vi "DAQmx Create Channel (CO-Pulse Generation-Frequency).vi"(0 "task in":refnum<k21>, 1 "frequency":dbl=1.0 format="%.6f", 2 "duty cycle":dbl=0.5 format="%.6f", 5 "counter":tag, 7 "name to assign":string, 9 "units":i32(ring)=10373 items=["Hz"=10373], 11 "error in":errorcluster, 12 "idle state":i32(ring)=10214 items=["High"=10192, "Low"=10214], 13 "initial delay":dbl format="%.6f") -> (4 "task out":refnum<k21>, 15 "error out":errorcluster)   [LabVIEW 2011]
doc: "Creates channel(s) to generate digital pulses that <B>frequency</B> and <B>duty cycle</B> define. The pulses appear on the default output terminal of the counter unless you select a different output terminal."
uses:
  C:/Program Files/National Instruments/LabVIEW 2011/resource/objmgr/daqmx.rc
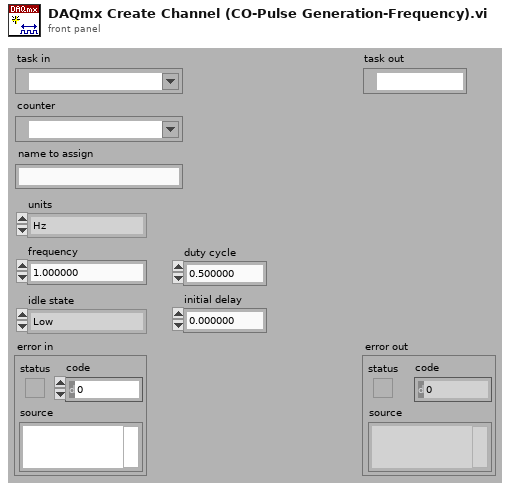
[diagram p1: front panel]
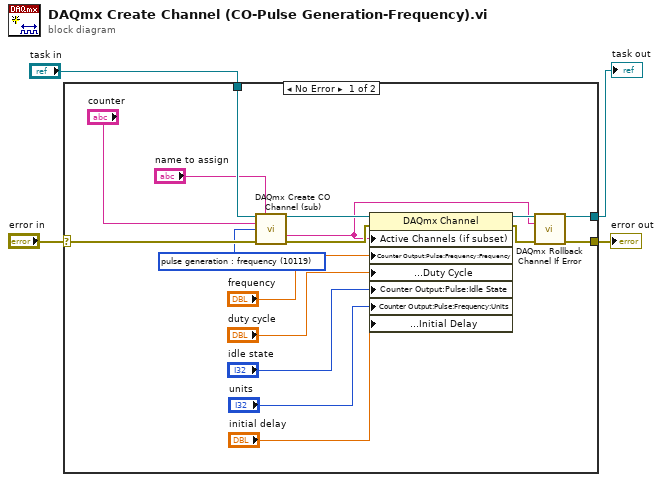
[diagram p0: block diagram]
diagram:
  n1 = case shown="No Error" "error in" {
    selector: "error in" -> [w19 w23]
    tunnel: [w6 w23] -> w3
    tunnel: "task in" -> [w21 w22]
    tunnel: [w7 w22] -> w1
    frame No Error {
      w13 = 10119 items=["pulse generation : frequency"=10119, "pulse generation : time"=10269, "pulse generation : ticks"=10268] ("output type")
      n2 = call "DAQmx Create CO Channel (sub).vi"("task in"=w21, "virtual channel name"="name to assign", "physical channel name"="counter", "output type"=w13, "error in"=w19) -> ("task out"=w11:refnum<k21>, "channel names"=w5:string, "error out"=w18:errorcluster)  [unwired: 8 out]
      n3 = property class="DAQmx Channel"(reference=w11, error in=w18, "Active Channels (if subset)"=w5, "Counter Output:Pulse:Frequency:Frequency"="frequency", "Counter Output:Pulse:Frequency:Duty Cycle"="duty cycle", "Counter Output:Pulse:Idle State"="idle state", "Counter Output:Pulse:Frequency:Units"="units", "Counter Output:Pulse:Frequency:Initial Delay"="initial delay") -> (reference out=w9:refnum<k21>, error out=w8:errorcluster)
      n4 = call "DAQmx Rollback Channel If Error.vi"("task in"=w9, "channel names"=w5, "error in"=w8) -> ("task out"=w7:refnum<k21>, "error out"=w6:errorcluster)  [unwired: 11 out]
    }
    frame Error {
    }
  }
  "error out" <- w3
  "task out" <- w1
